vi "qMVS.vi"(0 "System no.":i32=1 min=1 step=1, 2 "Axes to query":string[](array[string]), 3 "All axes?":bool, 4 "Axis identifier?":bool=TRUE, 5 "error in":errorcluster) -> (14 "Position values":dbl[](array[numeric]) format="%.6f", 15 "Step size":dbl[](array[numeric]) format="%.6f", 16 "Delay time (ms)":dbl[](array[numeric]), 19 "error out":errorcluster)   [LabVIEW 2026]
doc: "Returns last valid configuration for relative step move (caused by MVS) for the given axis.\nNote: The reported Step size may not be the last commanded value because during MVS the step size was automatically adapted so that the resulting number of steps is an integer value.\n\nC-702: If All axes? = TRUE, then Axis identifier? can be FALSE"
panel:
  # "Returns position information (actual or target position, depending\non system."
  # "If all axes: use"
  # "Query"
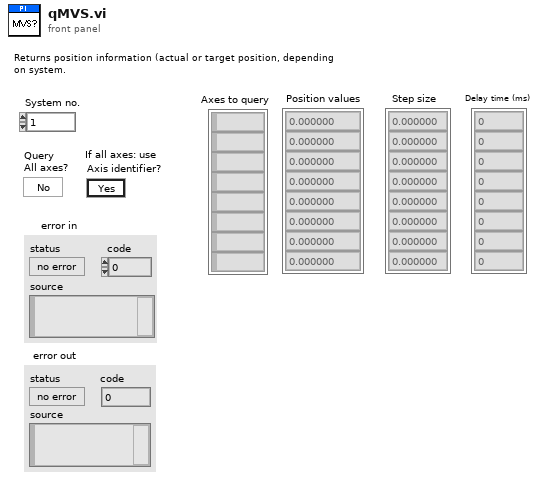
[diagram p1: front panel]
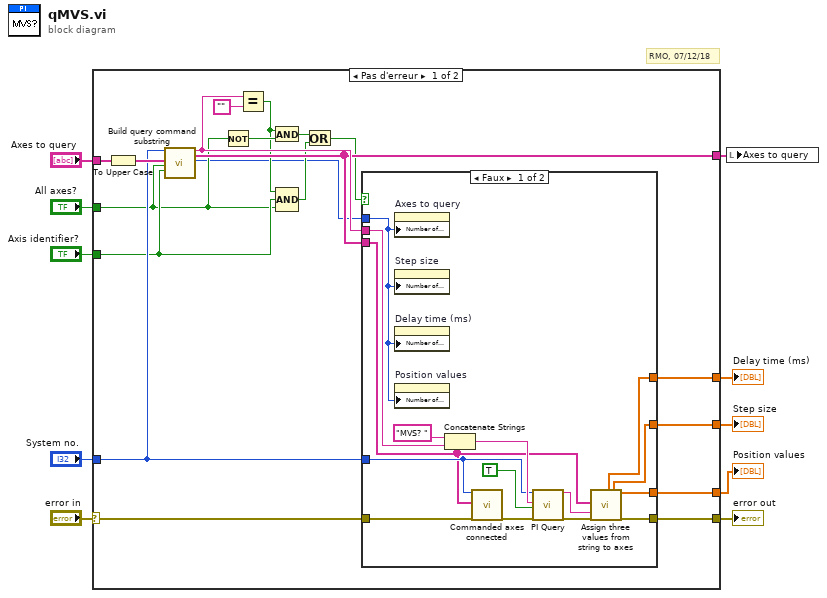
[diagram p0: block diagram]
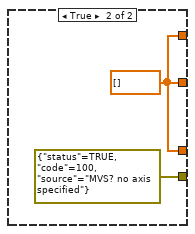
[diagram p2: hidden frame]
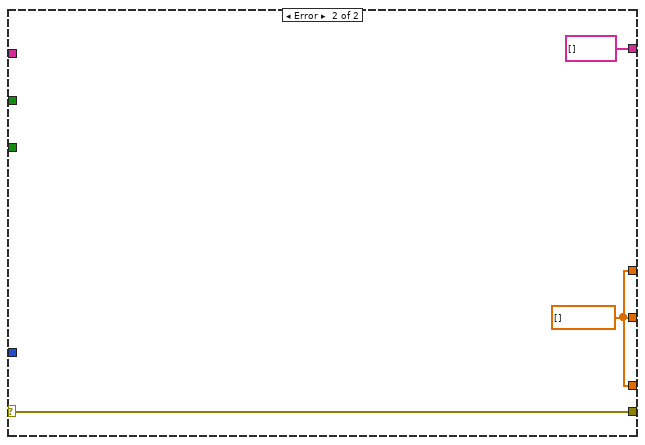
[diagram p3: hidden frame]
diagram:
  # "RMO, 07/12/18"
  n1 = case shown="Pas d'erreur" "error in" {
    selector: "error in" -> [w13 w47]
    tunnel: [w29 w48] -> w10
    tunnel: "Axes to query" -> [w28 _]
    tunnel: [w12 w47] -> w8
    tunnel: "System no." -> [w24 _]
    tunnel: [w23 string[] [] ("Axes to query out")] -> w6
    tunnel: "Axis identifier?" -> [w19 _]
    tunnel: "All axes?" -> [w18 _]
    tunnel: [w15 w48] -> w3
    tunnel: [w14 w48] -> w2
    frame No Error {
      n2 = To Upper Case(1:w28) -> (0:w26:string[])
      n3 = call "Build query command substring.vi"("System no."=w24, "Axes to query in"=w26, "Query\nAll axes?"=w18, "For all axes: use\nAxis identifier?"=w19) -> ("Command substring"=w25:string, "Axes to query out"=w23:string[], "Number of rows"=w16:u32)  [unwired: 2 in, 11 out]
      n4 = Not(x=w18) -> (.not. x?=w22:bool)
      n5 = Equal?(x=w25, y="" ("x")) -> (x = y?=w20:bool)
      n6 = And(x=w20, y=w22) -> (x .and. y?=w21:bool)
      n7 = Compound Arithmetic op=AND(w20, w19, w18) -> (w17:bool)
      n8 = Or(x=w21, y=w17) -> (x .or. y?=w11:bool)
      n9 = case shown="Faux" w11 {
        tunnel: [w41 w45] -> w29
        tunnel: w25 -> [w40 _]
        tunnel: w24 -> [w39 _]
        tunnel: w23 -> [w38 _]
        tunnel: w16 -> [w36 _]
        tunnel: [w35 w45] -> w15
        tunnel: [w34 w45] -> w14
        tunnel: w13 -> [w33 _]
        tunnel: [w30 errorcluster {"status"=TRUE, "code"=100, "source"="MVS? no axis specified"} ("error out")] -> w12
        frame False {
          n10 = property on="Axes to query" class="Tabl (strict)"("Number of Rows"=w36) -> ()  [unwired: 2 in, 2 out]
          n11 = property on="Step size" class="Tabl (strict)"("Number of Rows"=w36) -> ()  [unwired: 2 in, 2 out]
          n12 = property on="Delay time (ms)" class="Tabl (strict)"("Number of Rows"=w36) -> ()  [unwired: 2 in, 2 out]
          n13 = property on="Position values" class="Tabl (strict)"("Number of Rows"=w36) -> ()  [unwired: 2 in, 2 out]
          n14 = Concatenate Strings("MVS? ", w40) -> (w42:string)
          n15 = call "Commanded axes connected.vi"("System no."=w39, "Commanded axes"=w38, "error in"=w33) -> ("error out"=w37:errorcluster)  [unwired: 1 in, 15 out]
          n16 = call "PI Query.vi"("System no."=w39, "String to send"=w42, "Attach termination char.?"=TRUE ("Attach Linefeed?"), "error in"=w37) -> ("String read"=w31:string, "error out"=w32:errorcluster)  [unwired: 3 in, 11 out]
          n17 = call "Assign three values from string to axes.vi"("Queried axes"=w38, "Input String"=w31, "error in"=w32) -> ("Values 3"=w34:dbl[], "Values 2"=w35:dbl[], "Values 1"=w41:dbl[], "error out"=w30:errorcluster)  [unwired: 1 in, 12 out]
        }
        frame True {
          w45 = dbl[] [] ("Values 3")
        }
      }
    }
    frame Error {
      w48 = dbl[] [] ("Values")
    }
  }
  "error out" <- w8
  "Position values" <- w10
  "Step size" <- w3
  "Delay time (ms)" <- w2
  n18 = local write "Axes to query"(w6) -> ()
